vi "generate queues.vi"(8 "error in (no error)":errorcluster, 11 "Template in":refnum<class "Template.lvclass">) -> (0 "error out":errorcluster, 3 "Template out":refnum<class "Template.lvclass">)   [LabVIEW 2020, in "Template.lvlib" / "Template.lvclass"]
doc: "Creates the queues that will be used to control the actor's behavior.\nOverride this method if you need new queues in the application.\nCalling the parent method is <b>mandatory</b>\nThis vi is called in the Pre Launch Init override of the Actor Framework overrides."
uses:
  Template.lvclass
  Template.lvclass/Template.ctl
  typedefs/base actor queues.ctl
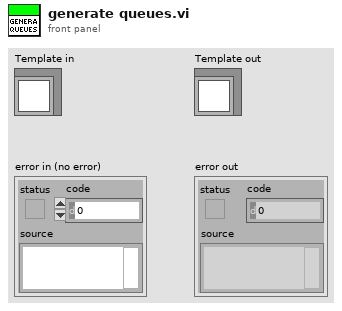
[diagram p1: front panel]
types:
  T1 = typedef "Template.lvlib/Template.lvclass/base actor queues.ctl" = cluster{"DVR Pool":refnum<queue>, "Actor's Data":refnum<queue>}
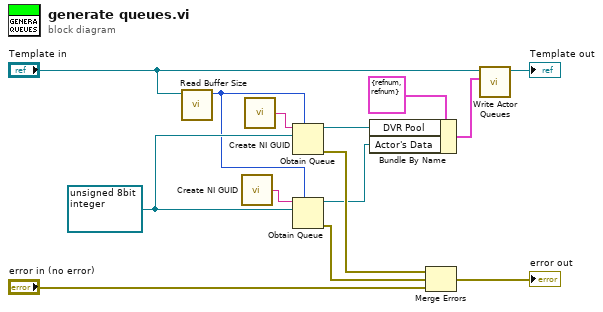
[diagram p0: block diagram]
diagram:
  w2 = refnum<data-value> refnum ("Data Value Refnum")
  n1 = call "Read Buffer Size.vi"("Template in"="Template in") -> ("DVR Pool Size"=w1:i32)  [unwired: 10 in]
  n2 = call <vilib>:"Create NI GUID.vi"() -> ("NI GUID"=w8:string)
  n3 = call <vilib>:"Create NI GUID.vi"() -> ("NI GUID"=w11:string)
  n4 = Obtain Queue(max queue size (-1, unlimited)=w1, name (unnamed)=w11, element data type=w2) -> (queue out=w3:refnum<queue>, error out=w9:errorcluster)  [unwired: 2 in, 1 out]
  n5 = Obtain Queue(max queue size (-1, unlimited)=w1, name (unnamed)=w8, element data type=w2) -> (queue out=w5:refnum<queue>, error out=w4:errorcluster)  [unwired: 2 in, 1 out]
  n6 = Bundle By Name(cluster=T1 {"DVR Pool"=refnum, "Actor's Data"=refnum} ("Base Actor Queues"), "DVR Pool"=w3, "Actor's Data"=w5) -> (w6:T1)
  n7 = Merge Errors(w9, w4, "error in (no error)") -> (→"error out":errorcluster)
  n8 = call "Write Actor Queues.vi"("Base Actor Queues"=w6, "Template in"="Template in") -> ("Template out"=→"Template out":refnum<class "Template.lvclass">)  [unwired: 9 in]
